vi "Port.vi"(8 "error in (no error)":errorcluster, 11 "Node Ptr":T1 format="%.0x") -> (0 "error out":errorcluster)   [LabVIEW 2017, in "NI-XNET Monitor System Explorer.lvlib"]
uses:
  NI-XNET Monitor System Explorer.lvlib
  <vilib>/NI Veristand/Custom Device API/Custom Device Item Ref.ctl
  <vilib>/NI Veristand/Custom Device API/Get Item Property (I32).vi
  Shared/Constants.vi
  <vilib>/NI Veristand/Custom Device API/Get Item Property (String).vi
  <vilib>/NI Veristand/Custom Device API/Get Item Property (Boolean).vi
  <vilib>/NI Veristand/Custom Device API/Set Item Property (Boolean).vi
  <vilib>/NI Veristand/Custom Device API/Custom Device API.lvlib
  Shared/NI-XNET Monitor Shared.lvlib
  <vilib>/NI VeriStand/Custom Device Tools/Custom Device Utility Library/Custom Device Utility Library.lvlib
panel:
  out "Info Cluster":cluster{"String":string}={"String"="This port is disabled under the NI-XNET hardware configuration section. Go to the port definition to enable it."}
  in  "GoTo":bool
  in  "Force Disable Port Monitor":bool
  out "NI-XNET Port (SDF Path)":string
  out "Port Address":string
  in  "Header":cluster{"Section Name":string}={"Section Name"=" Port Settings"}
  in  "Description":string
  out "Port Name":string
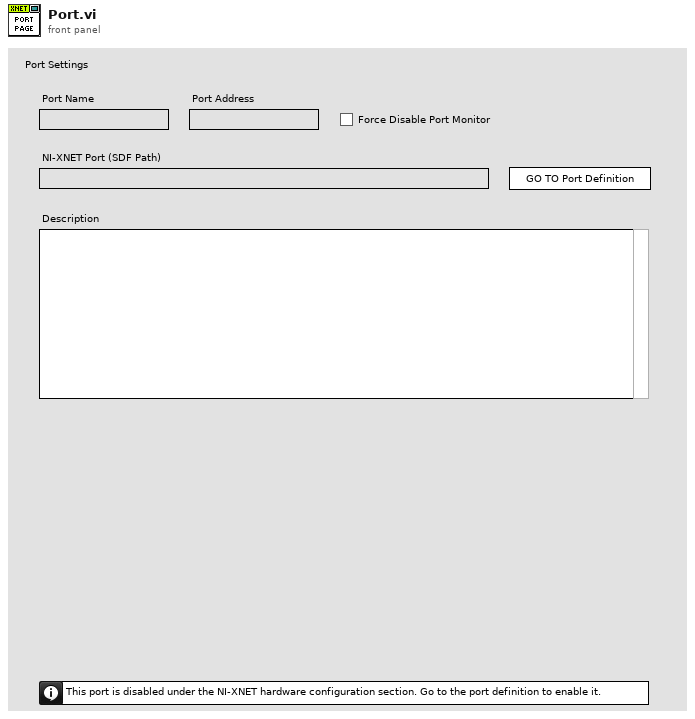
[diagram p1: front panel]
types:
  T1 = typedef "Custom Device API.lvlib/Custom Device Item Ref.ctl" = u64
  T2 = typedef "Custom Device API.lvlib/Custom Device Item Info.ctl" = cluster{"Name":string, "Is Channel":bool, "GUID":string, "Is Waveform":bool}
  T3 = typedef "Custom Device API.lvlib/Custom Device Commands.ctl" = enum16{"Default", "Item renamed", "Shutdown", "Dynamic button pressed"}
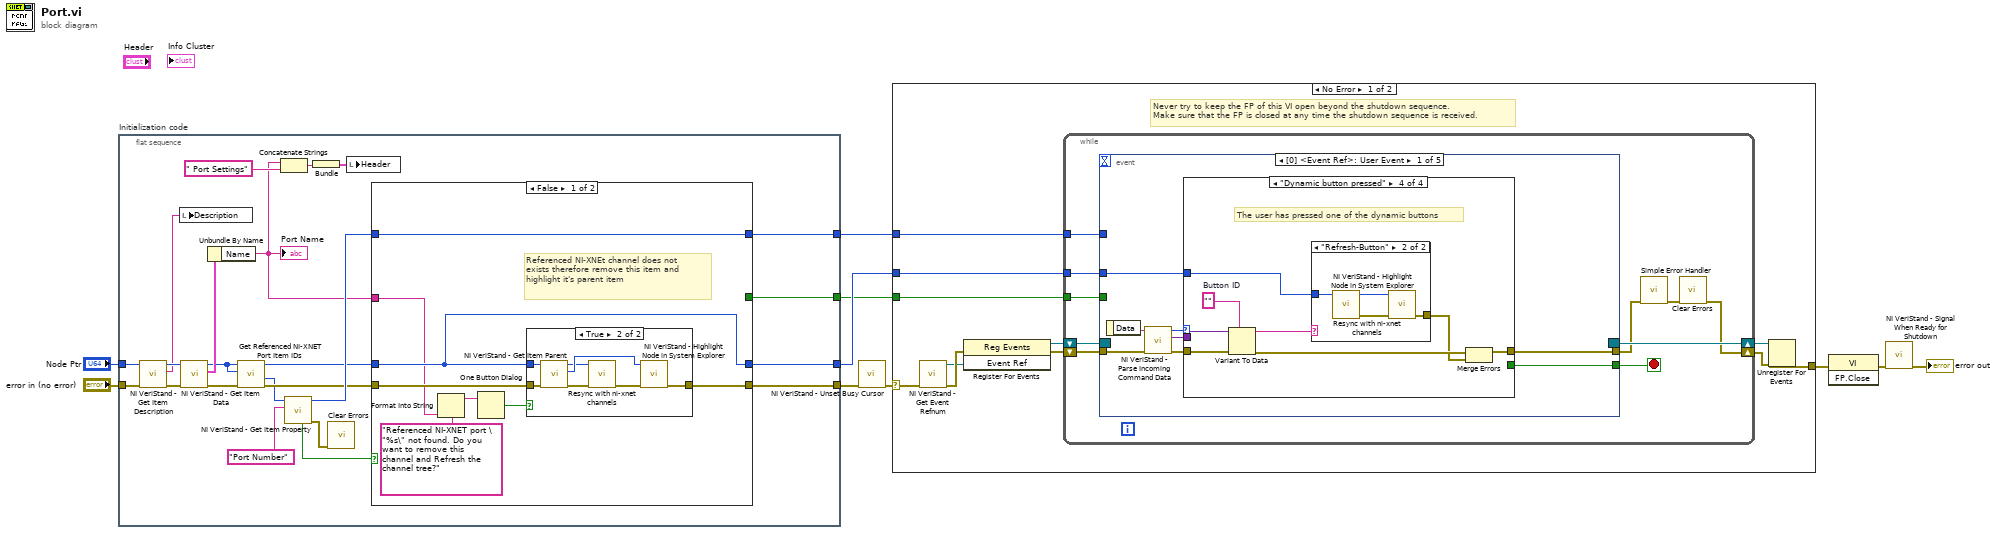
[diagram p0: block diagram]
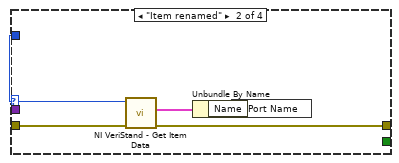
[diagram p3: hidden frame]
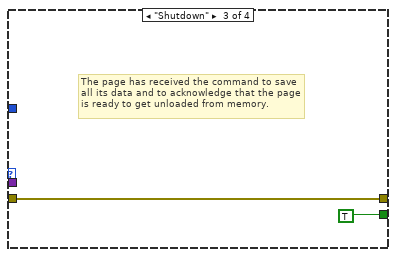
[diagram p4: hidden frame]
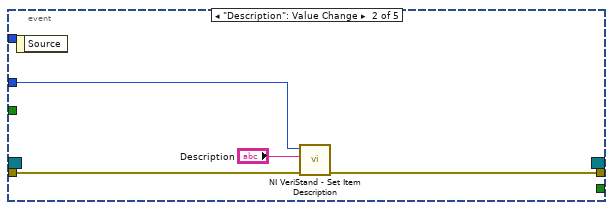
[diagram p6: hidden frame]
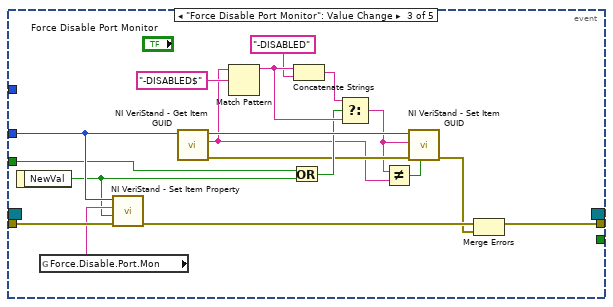
[diagram p7: hidden frame]
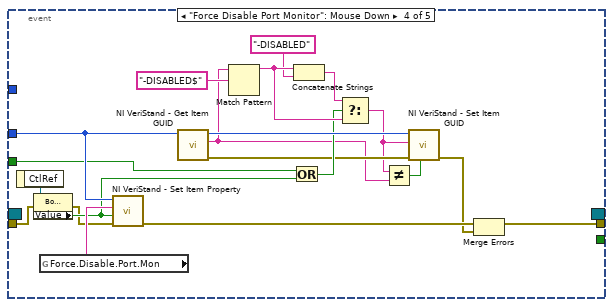
[diagram p8: hidden frame]
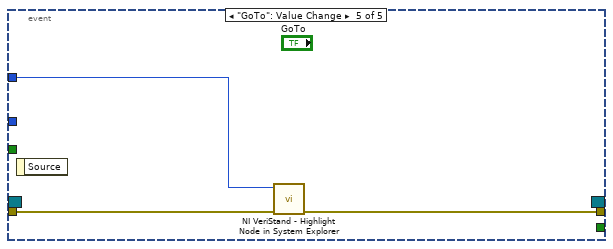
[diagram p9: hidden frame]
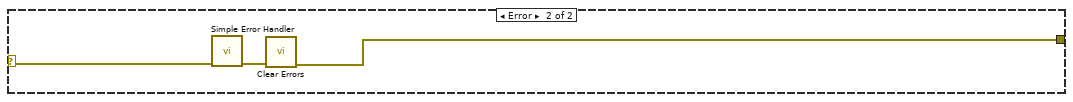
[diagram p10: hidden frame]
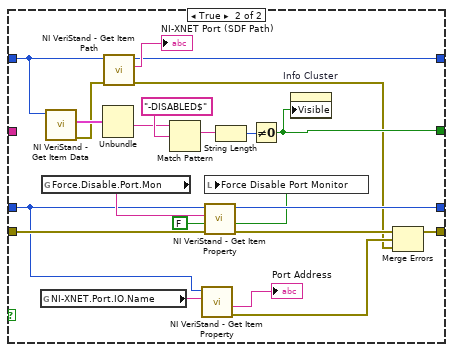
[diagram p12: hidden frame]
diagram:
  n1 = flat-sequence "Initialization code" {
    tunnel: "error in (no error)" -> [w32]
    tunnel: "Node Ptr" -> [w31]
    tunnel: [w25] -> w4
    tunnel: [w24] -> w3
    tunnel: [w26] -> w2
    tunnel: [w22] -> w1
    frame #0 {
      n2 = call <vilib>:"NI VeriStand - Get Item Description.vi"("error in (no error)"=w32, "Item Ref in"=w31) -> ("error out"=w29:errorcluster, "Description"=w30:string, "Item Ref out"=w33:T1)  [unwired: 7 out]
      n3 = local write "Description"(w30) -> ()
      n4 = call <vilib>:"NI VeriStand - Get Item Data.vi"("error in (no error)"=w29, "Item Ref in"=w33) -> ("error out"=w18:errorcluster, "Item Info"=w28:T2, "Item Ref out"=w16:T1)  [unwired: 7 out]
      n5 = Unbundle By Name(w28) -> ("Name"=w11:string)
      "Port Name" <- w11
      n6 = call "Get Referenced NI-XNET Port Item IDs.vi"("Error In"=w18, "CD Port Item Ref In"=w16, "Device Item Ref in in"=w16) -> ("Error Out"=w17:errorcluster, "NI-XNET Port Item Ref Out"=w15:T1, "Device Item Ref out"=w19:T1)  [unwired: 5 in, 1 out]
      n7 = Concatenate Strings(w11, " Port Settings" ("Section Name")) -> (w13:string)
      n8 = call-poly <vilib>:"NI VeriStand - Get Item Property.vi"("Property Name"="Port Number", "Item Ref in"=w15) -> ("error out"=w21:errorcluster, "Item Ref out"=w20:T1, "Found?"=w23:bool)  [unwired: 6 in, 1 out]
      n9 = Bundle(w13) -> (w14:cluster{string})  [unwired: 1 in]
      n10 = call <vilib>:"Clear Errors.vi"("error in (no error)"=w21) -> ()  [unwired: 5 in, 2 out]
      n11 = local write "Header"(w14) -> ()
      n12 = case shown="False" w23 {
        tunnel: w17 -> [w41 w55]
        tunnel: [w40 w54] -> w26
        tunnel: w19 -> [w38 w50]
        tunnel: [w38 w65] -> w25
        tunnel: [_ w62] -> w24
        tunnel: w20 -> [w39 w57]
        tunnel: [w39 w60] -> w22
        tunnel: w11 -> [w35 _]
        frame False {
          # "Referenced NI-XNEt channel does not exists therefore remove this item and highlight it's parent item"
          n13 = Format Into String(format string="Referenced NI-XNET port \"%s\" not found. Do you want to remove this channel and Refresh the channel tree?", w35) -> (resulting string=w36:string)  [unwired: 2 in, 1 out]
          n14 = One Button Dialog(message=w36) -> (true=w37:bool)  [unwired: 1 in]
          n15 = case shown="True" w37 {
            tunnel: w41 -> [w42 w49]
            tunnel: [w42 w48] -> w40
            tunnel: w38 -> [_ w47]
            frame False {
            }
            frame True {
              n16 = call <vilib>:"NI VeriStand - Get Item Parent.vi"("error in (no error)"=w49, "Item Ref in"=w47) -> ("error out"=w44:errorcluster, "Parent Ref"=w46:T1, "Item Ref out"=w45:T1)  [unwired: 6 in, 1 out]
              n17 = call "Resync with ni-xnet channels.vi"("Error In"=w44, "Device Item Ref in in"=w45) -> ("Error Out"=w43:errorcluster)  [unwired: 8 in, 1 out]
              n18 = call <vilib>:"NI VeriStand - Highlight Node in System Explorer.vi"("error in (no error)"=w43, "Item Ref in"=w46) -> ("error out"=w48:errorcluster)  [unwired: 8 in, 1 out]
            }
          }
        }
        frame True {
          n19 = global read "Constants.vi" "NI-XNET.Port.IO.Name"() -> (w59:string)
          n20 = global read "Constants.vi" "Force.Disable.Port.Mon"() -> (w66:string)
          n21 = call <vilib>:"NI VeriStand - Get Item Data.vi"("Item Ref in"=w57) -> ("error out"=w52:errorcluster, "Item Info"=w71:T2)  [unwired: 7 in, 2 out]
          n22 = Unbundle(w71) -> ("GUID"=w69:string)  [unwired: 3 out]
          n23 = call <vilib>:"NI VeriStand - Get Item Path.vi"("error in (no error)"=w52, "Item Ref in"=w57) -> ("error out"=w51:errorcluster, "Path"=→"NI-XNET Port (SDF Path)":string, "Item Ref out"=w60:T1)  [unwired: 6 in, 1 out]
          n24 = Match Pattern(string=w69, regular expression="-DISABLED$") -> (match substring=w68:string)  [unwired: 1 in, 3 out]
          n25 = call-poly <vilib>:"NI VeriStand - Get Item Property.vi"("Property Name"=w59, "Item Ref in"=w50) -> ("error out"=w58:errorcluster, "Value"=→"Port Address":string)  [unwired: 6 in, 2 out]
          n26 = call-poly <vilib>:"NI VeriStand - Get Item Property.vi"("error in (no error)"=w55, "Default Value"=FALSE, "Property Name"=w66, "Item Ref in"=w50) -> ("error out"=w53:errorcluster, "Value"=w63:bool, "Item Ref out"=w65:T1)  [unwired: 4 in, 1 out]
          n27 = local write "Force Disable Port Monitor"(w63) -> ()
          n28 = String Length(string=w68) -> (length=w67:i32)
          n29 = Not Equal To 0?(x=w67) -> (x != 0?=w62:bool)
          n30 = property on="Info Cluster" class="Clust (strict)"("Visible"=w62) -> ()  [unwired: 2 in, 2 out]
          n31 = Merge Errors(w53, w58, w51) -> (w54:errorcluster)
        }
      }
    }
  }
  n32 = call <vilib>:"NI VeriStand - Unset Busy Cursor.vi"("error in (no error)"=w2) -> ("error out"=w6:errorcluster)  [unwired: 10 out]
  n33 = case shown="No Error" w6 {
    selector: w6 -> [w75 w168]
    tunnel: [w79 w166] -> w10
    tunnel: w4 -> [w73 _]
    tunnel: w3 -> [w74 _]
    tunnel: w1 -> [w72 _]
    frame No Error {
      # "Never try to keep the FP of this VI open beyond the shutdown sequence.\nMake sure that the FP is closed at any time the shutdown sequence is received."
      n34 = call <vilib>:"NI VeriStand - Get Event Refnum.vi"("error in (no error)"=w75) -> ("error out"=w82:errorcluster, "Event Ref"=w78:refnum<user-event>)  [unwired: 9 out]
      n35 = register-events(error in=w82, w78) -> (reference out=w76:refnum<event-registration>, error out=w77:errorcluster)  [unwired: 1 in]
      n36 = while {
        tunnel: w73 -> [w88]
        shift-right: [w85] -> w80
        shift-left: w77 -> [w91]
        shift-right: [w92] -> w81
        shift-left: w76 -> [w90]
        tunnel: w74 -> [w84]
        tunnel: w72 -> [w83]
        stop <- w89 stop-if-true
        n37 = event shown="[0] <Event Ref>: User Event" {
          selector: w90 -> [_ _ _ _ _]
          dyn-events: [_ _ _ _ _] -> w92
          timeout: _ -> [_ _ _ _ _]
          tunnel: w91 -> [w100 w123 w142 w143 w164]
          tunnel: [w96 _ _ _ _] -> w89
          tunnel: [w95 w122 w135 w157 w163] -> w87
          tunnel: w88 -> [w94 w124 w139 w160 _]
          tunnel: w84 -> [_ _ w128 w150 _]
          tunnel: w83 -> [_ _ _ _ w165]
          event User Event {
            n38 = event-data() -> ("Data"=w99:string)  [unwired: 1 out]
            n39 = call <vilib>:"NI VeriStand - Parse Incoming Command Data.vi"("error in (no error)"=w100, "Incoming data"=w99) -> ("error out"=w98:errorcluster, "Outgoing data"=w93:variant, "Action"=w97:T3)  [unwired: 7 out]
            n40 = case shown="\"Dynamic button pressed\"" w97 {
              tunnel: w98 -> [w101 w106 w107 w116]
              tunnel: [_ _ TRUE _] -> w96
              tunnel: [w101 w103 w107 w110] -> w95
              tunnel: w94 -> [_ w105 _ w111]
              tunnel: w93 -> [_ _ _ w115]
              frame "Default", Default {
              }
              frame "Item renamed" {
                n41 = call <vilib>:"NI VeriStand - Get Item Data.vi"("error in (no error)"=w106, "Item Ref in"=w105) -> ("error out"=w103:errorcluster, "Item Info"=w104:T2)  [unwired: 8 out]
                n42 = Unbundle By Name(w104) -> ("Name"=w102:string)
                n43 = local write "Port Name"(w102) -> ()
              }
              frame "Shutdown" {
                # "The page has received the command to save all its data and to acknowledge that the page is ready to get unloaded from memory."
              }
              frame "Dynamic button pressed" {
                w114 = ""  # Button ID
                # "The user has pressed one of the dynamic buttons"
                n44 = Variant To Data(error in=w116, type=w114, Variant=w115) -> (data=w112:string, error out=w113:errorcluster)
                n45 = case shown="\"Refresh-Button\"" w112 {
                  tunnel: w111 -> [_ w120]
                  tunnel: [_ w117] -> w109
                  frame Default {
                  }
                  frame "Refresh-Button" {
                    n46 = call "Resync with ni-xnet channels.vi"("Device Item Ref in in"=w120) -> ("Error Out"=w118:errorcluster, "Device Item Ref out"=w119:T1)  [unwired: 9 in]
                    n47 = call <vilib>:"NI VeriStand - Highlight Node in System Explorer.vi"("error in (no error)"=w118, "Item Ref in"=w119) -> ("error out"=w117:errorcluster)  [unwired: 8 in, 1 out]
                  }
                }
                n48 = Merge Errors(w113, w109) -> (w110:errorcluster)
              }
            }
          }
          event "Description": Value Change {
            n49 = event-data() -> ()  [unwired: 2 out]
            n50 = call <vilib>:"NI VeriStand - Set Item Description.vi"("error in (no error)"=w123, "Description"="Description", "Item Ref in"=w124) -> ("error out"=w122:errorcluster)  [unwired: 8 out]
          }
          event "Force Disable Port Monitor": Value Change {
            n51 = event-data() -> ("NewVal"=w136:bool)  [unwired: 1 out]
            n52 = global read "Constants.vi" "Force.Disable.Port.Mon"() -> (w140:string)
            n53 = call-poly <vilib>:"NI VeriStand - Set Item Property.vi"("error in (no error)"=w142, "Value"=w136, "Property Name"=w140, "Item Ref in"=w139) -> ("error out"=w141:errorcluster)  [unwired: 5 in, 2 out]
            n54 = call <vilib>:"NI VeriStand - Get Item GUID.vi"("Item Ref in"=w139) -> ("error out"=w129:errorcluster, "GUID"=w125:string, "Item Ref out"=w138:T1)  [unwired: 8 in]
            n55 = Match Pattern(string=w125, regular expression="-DISABLED$") -> (before substring=w132:string)  [unwired: 1 in, 3 out]
            n56 = Or(x=w128, y=w136) -> (x .or. y?=w130:bool)
            n57 = Concatenate Strings(w132, "-DISABLED" ("regular expression")) -> (w133:string)
            n58 = Select(t=w133, s=w130, f=w132) -> (s? t:f=w126:string)
            n59 = Not Equal?(x=w126, y=w125) -> (x != y?=w127:bool)
            n60 = call <vilib>:"NI VeriStand - Set Item GUID.vi"("Refresh System Explorer Tree? (F)"=w127, "error in (no error)"=w129, "GUID"=w126, "Item Ref in"=w138) -> ("error out"=w134:errorcluster)  [unwired: 6 in, 1 out]
            n61 = Merge Errors(w141, w134) -> (w135:errorcluster)
          }
          event "Force Disable Port Monitor": Mouse Down {
            n62 = event-data() -> ("CtlRef"=w146:refnum<vi>)  [unwired: 1 out]
            n63 = property class="Bool (strict)"(reference=w146, error in=w143) -> (error out=w144:errorcluster, "Value"=w145:bool)  [unwired: 1 out]
            n64 = global read "Constants.vi" "Force.Disable.Port.Mon"() -> (w161:string)
            n65 = call-poly <vilib>:"NI VeriStand - Set Item Property.vi"("error in (no error)"=w144, "Value"=w145, "Property Name"=w161, "Item Ref in"=w160) -> ("error out"=w162:errorcluster)  [unwired: 5 in, 2 out]
            n66 = call <vilib>:"NI VeriStand - Get Item GUID.vi"("Item Ref in"=w160) -> ("error out"=w151:errorcluster, "GUID"=w147:string, "Item Ref out"=w159:T1)  [unwired: 8 in]
            n67 = Match Pattern(string=w147, regular expression="-DISABLED$") -> (before substring=w154:string)  [unwired: 1 in, 3 out]
            n68 = Or(x=w150, y=w145) -> (x .or. y?=w152:bool)
            n69 = Concatenate Strings(w154, "-DISABLED" ("regular expression")) -> (w155:string)
            n70 = Select(t=w155, s=w152, f=w154) -> (s? t:f=w148:string)
            n71 = Not Equal?(x=w148, y=w147) -> (x != y?=w149:bool)
            n72 = call <vilib>:"NI VeriStand - Set Item GUID.vi"("Refresh System Explorer Tree? (F)"=w149, "error in (no error)"=w151, "GUID"=w148, "Item Ref in"=w159) -> ("error out"=w156:errorcluster)  [unwired: 6 in, 1 out]
            n73 = Merge Errors(w162, w156) -> (w157:errorcluster)
          }
          event "GoTo": Value Change {
            n74 = event-data() -> ()  [unwired: 2 out]
            n75 = call <vilib>:"NI VeriStand - Highlight Node in System Explorer.vi"("error in (no error)"=w164, "Item Ref in"=w165) -> ("error out"=w163:errorcluster)  [unwired: 8 in, 1 out]
          }
        }
        n76 = call <vilib>:"Simple Error Handler.vi"("error in (no error)"=w87) -> ("error out"=w86:errorcluster)  [unwired: 1 in, 7 out]
        n77 = call <vilib>:"Clear Errors.vi"("error in (no error)"=w86) -> ("error out"=w85:errorcluster)  [unwired: 1 in, 5 out]
      }
      n78 = Unregister For Events(event registration refnum=w81, error in=w80) -> (error out=w79:errorcluster)
    }
    frame Error {
      n79 = call <vilib>:"Simple Error Handler.vi"("error in (no error)"=w168) -> ("error out"=w167:errorcluster)  [unwired: 1 in, 7 out]
      n80 = call <vilib>:"Clear Errors.vi"("error in (no error)"=w167) -> ("error out"=w166:errorcluster)  [unwired: 1 in, 5 out]
    }
  }
  n81 = invoke class="VI" method="FP.Close"(error in=w10) -> (error out=w9:errorcluster)  [unwired: 2 in, 2 out]
  n82 = call <vilib>:"NI VeriStand - Signal When Ready for Shutdown.vi"("error in (no error)"=w9) -> ("error out"=→"error out":errorcluster)  [unwired: 10 out]
